vi "oldProceed.vi"(8 "error in (no error)":errorcluster, 11 "DAQMH121119OrcaFlash in":refnum<class "DAQOrcaFlash.lvclass">) -> (0 "error out":errorcluster, 3 "DAQMH121119OrcaFlash out":refnum<class "DAQOrcaFlash.lvclass">)   [LabVIEW 2012]
uses:
  DAQOrcaFlash.lvclass
  Murmex/LabVIEW/Murmex/Murmex/Murmex.lvclass
  Murmex/LabVIEW/Murmex/StopMessage/StopMessage.lvclass
  Murmex/LabVIEW/Murmex/GenericMessage/GenericMessage.lvclass
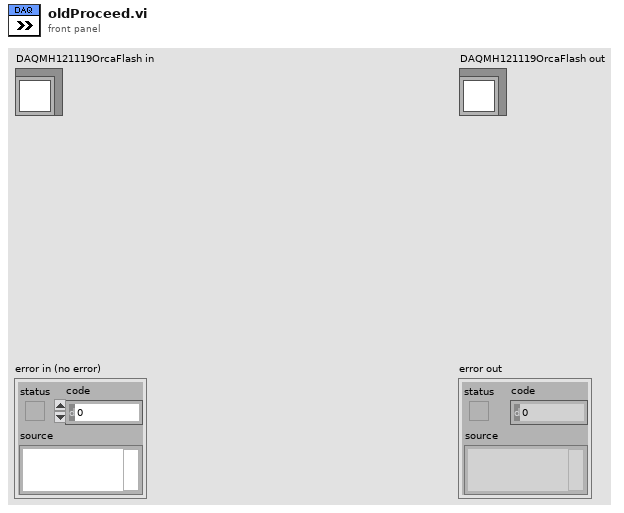
[diagram p1: front panel]
types:
  T1 = typedef "DAQOrcaFlash.lvclass/imaging_mode.ctl" = enum16{"focus mode", "single sweep"}
  T2 = typedef "IMAQ Image.ctl" = refnum<image>
  T3 = cluster{"width":u32, "height":u32, "datatype":u32}
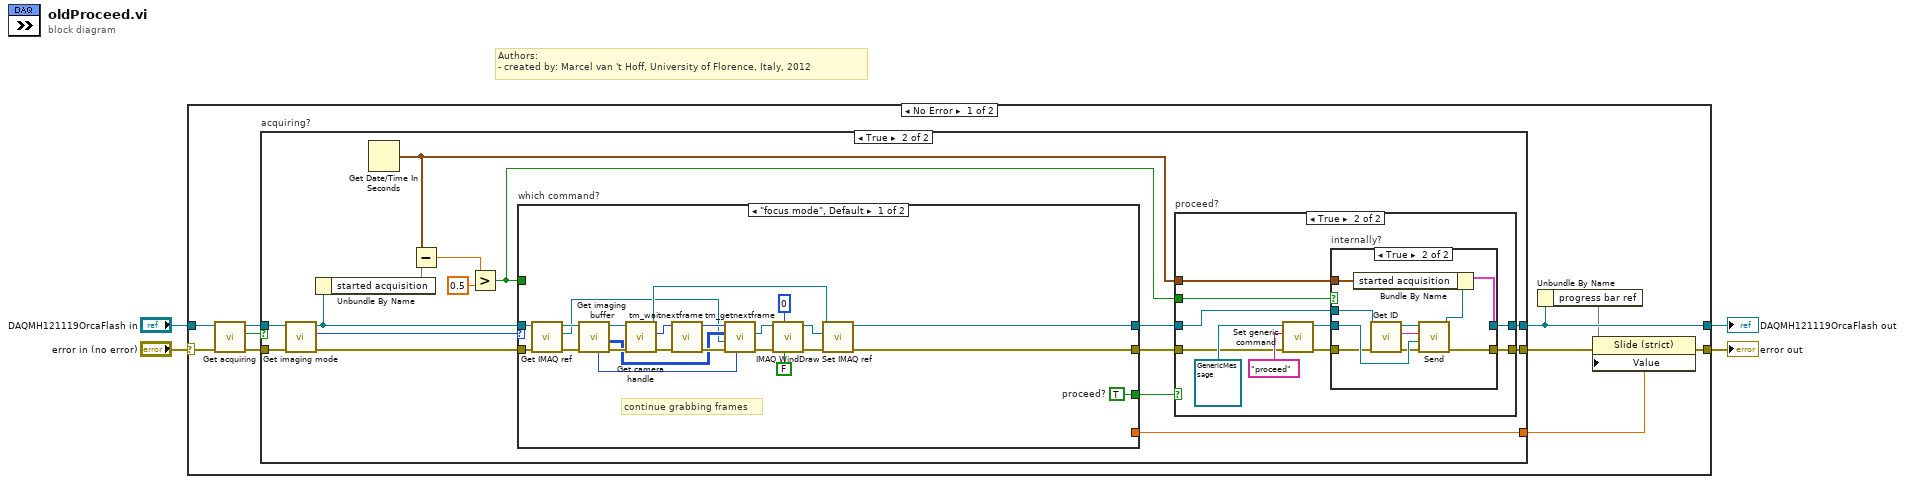
[diagram p0: block diagram]
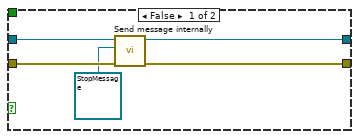
[diagram p3: hidden frame]
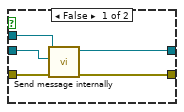
[diagram p4: hidden frame]
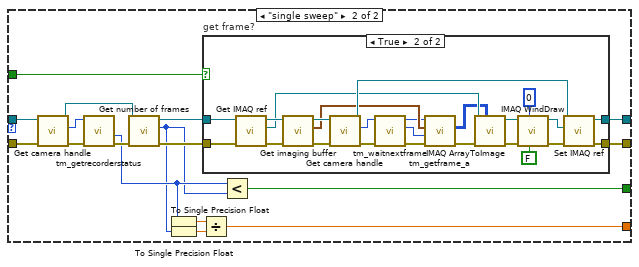
[diagram p5: hidden frame]
diagram:
  # "Authors: \n- created by: Marcel van 't Hoff, University of Florence, Italy, 2012"
  n1 = case shown="No Error" "error in (no error)" {
    selector: "error in (no error)" -> [w12 w130]
    tunnel: [w6 w130] -> w3
    tunnel: [w9 w129] -> w1
    tunnel: "DAQMH121119OrcaFlash in" -> [w14 w129]
    frame No Error {
      n2 = call "Get acquiring.vi"("error in (no error)"=w12, "DAQMH121119OrcaFlash in"=w14) -> ("error out"=w11:errorcluster, "is acquiring?"=w10:bool, "DAQMH121119OrcaFlash out"=w13:refnum<class "DAQOrcaFlash.lvclass">)  [unwired: 7 in]
      n3 = case "acquiring?" shown="True" w10 {
        tunnel: [w15 w24] -> w5
        tunnel: [w16 w25] -> w9
        tunnel: w13 -> [w16 w30]
        tunnel: w11 -> [w15 w29]
        tunnel: [_ w28] -> w7
        frame False {
        }
        frame True {
          n4 = call "Get imaging mode.vi"("error in (no error)"=w29, "DAQMH121119OrcaFlash in"=w30) -> ("error out"=w32:errorcluster, "imaging mode"=w31:T1, "DAQMH121119OrcaFlash out"=w18:refnum<class "DAQOrcaFlash.lvclass">)  [unwired: 7 in]
          n5 = Unbundle By Name(w18) -> ("started acquisition"=w20)
          n6 = Get Date/Time In Seconds() -> (seconds since 1Jan1904=w17:timestamp)
          n7 = Subtract(x=w17, y=w20) -> (x-y=w21:dbl)
          n8 = Greater?(x=w21, y=0.5) -> (0:w19:bool)
          n9 = case "which command?" shown="\"focus mode\", Default" w31 {
            tunnel: w32 -> [w84 w102]
            tunnel: w18 -> [w85 w100]
            tunnel: [w83 w90] -> w27
            tunnel: [w82 w91] -> w26
            tunnel: [_ w92] -> w28
            tunnel: [w81 w86] -> w23
            tunnel: w19 -> [_ w89]
            frame "focus mode", Default {
              w81 = TRUE  # proceed?
              # "continue grabbing frames"
              n10 = call "Get IMAQ ref.vi"("error in (no error)"=w84, "DAQMH121119OrcaFlash in"=w85) -> ("error out"=w74:errorcluster, "IMAQ reference"=w70:T2, "DAQMH121119OrcaFlash out"=w77:refnum<class "DAQOrcaFlash.lvclass">)  [unwired: 7 in]
              n11 = call "Get imaging buffer.vi"("error in (no error)"=w74, "DAQMH121119OrcaFlash in"=w77) -> ("error out"=w73:errorcluster, "Buffer 2"=w71:u16[][], "DAQMH121119OrcaFlash out"=w75:refnum<class "DAQOrcaFlash.lvclass">, "Image type"=w69:u32)  [unwired: 5 in, 1 out]
              n12 = call "Get camera handle.vi"("error in (no error)"=w73, "DAQMH121119OrcaFlash in"=w75) -> ("error out"=w78:errorcluster, "cam handle"=w79:u32, "DAQMH121119OrcaFlash out"=w76:refnum<class "DAQOrcaFlash.lvclass">)  [unwired: 7 in]
              n13 = call <userlib>:"tm_waitnextframe.vi"("error in (no error)"=w78, "Handle in"=w79) -> ("error out"=w80:errorcluster, "Handle out"=w72:u32)  [unwired: 6 in, 2 out]
              n14 = call <userlib>:"tm_getnextframe.vi"("Image Type"=w69, "error in (no error)"=w80, "Image"=w70, "Buffer"=w71, "Handle in"=w72) -> ("error out"=w66:errorcluster, "New Image"=w68:T2)  [unwired: 4 in, 1 out]
              n15 = call "IMAQ WindDraw"("Resize to Image Size? (Y)"=FALSE, "Window Number (0...15)"=0, "error in (no error)"=w66, "Image"=w68) -> ("error out"=w65:errorcluster, "Image Out (duplicate)"=w67:T2)  [unwired: 6 in]
              n16 = call "Set IMAQ ref.vi"("error in (no error)"=w65, "IMAQ reference"=w67, "DAQMH121119OrcaFlash in"=w76) -> ("error out"=w83:errorcluster, "DAQMH121119OrcaFlash out"=w82:refnum<class "DAQOrcaFlash.lvclass">)  [unwired: 7 in]
            }
            frame "single sweep" {
              n17 = call "Get camera handle.vi"("error in (no error)"=w102, "DAQMH121119OrcaFlash in"=w100) -> ("error out"=w101:errorcluster, "cam handle"=w99:u32, "DAQMH121119OrcaFlash out"=w98:refnum<class "DAQOrcaFlash.lvclass">)  [unwired: 7 in]
              n18 = call <userlib>:"tm_getrecorderstatus.vi"("error in (no error)"=w101, "Handle"=w99) -> ("error out"=w97:errorcluster, "Count"=w88:i32)  [unwired: 6 in, 2 out]
              n19 = call "Get number of frames.vi"("error in (no error)"=w97, "DAQMH121119OrcaFlash in"=w98) -> ("error out"=w96:errorcluster, "no. of frames"=w87:i32, "DAQMH121119OrcaFlash out"=w95:refnum<class "DAQOrcaFlash.lvclass">)  [unwired: 7 in]
              n20 = To Single Precision Float(number=w88) -> (single precision float=w93:sgl)
              n21 = To Single Precision Float(number=w87) -> (single precision float=w94:sgl)
              n22 = Divide(x=w93, y=w94) -> (x/y=w92:sgl)
              n23 = case "get frame?" shown="True" w89 {
                tunnel: w96 -> [w104 w120]
                tunnel: w95 -> [w103 w119]
                tunnel: [w103 w117] -> w91
                tunnel: [w104 w118] -> w90
                frame False {
                }
                frame True {
                  n24 = call "Get IMAQ ref.vi"("error in (no error)"=w120, "DAQMH121119OrcaFlash in"=w119) -> ("error out"=w127:errorcluster, "IMAQ reference"=w122:T2, "DAQMH121119OrcaFlash out"=w124:refnum<class "DAQOrcaFlash.lvclass">)  [unwired: 7 in]
                  n25 = call "Get imaging buffer.vi"("error in (no error)"=w127, "DAQMH121119OrcaFlash in"=w124) -> ("error out"=w128:errorcluster, "imaging buffer"=w116:T3, "DAQMH121119OrcaFlash out"=w126:refnum<class "DAQOrcaFlash.lvclass">)  [unwired: 5 in, 2 out]
                  n26 = call "Get camera handle.vi"("error in (no error)"=w128, "DAQMH121119OrcaFlash in"=w126) -> ("error out"=w112:errorcluster, "cam handle"=w115:u32, "DAQMH121119OrcaFlash out"=w125:refnum<class "DAQOrcaFlash.lvclass">)  [unwired: 7 in]
                  n27 = call <userlib>:"tm_waitnextframe.vi"("error in (no error)"=w112, "Handle in"=w115) -> ("error out"=w111:errorcluster, "Frame Index"=w113:i32, "Handle out"=w114:u32)  [unwired: 6 in, 1 out]
                  n28 = call <userlib>:"tm_getframe_a.vi"("error in (no error)"=w111, "Frame Index"=w113, "Buffer"=w116, "Handle in"=w114) -> ("error out"=w123:errorcluster, "Data 16"=w121:u16[][])  [unwired: 3 in, 3 out]
                  n29 = call "IMAQ ArrayToImage"("Image Pixels (U16)"=w121, "error in (no error)"=w123, "Image"=w122) -> ("error out"=w110:errorcluster, "Image Out"=w108:T2)  [unwired: 7 in]
                  n30 = call "IMAQ WindDraw"("Resize to Image Size? (Y)"=FALSE, "Window Number (0...15)"=0, "error in (no error)"=w110, "Image"=w108) -> ("error out"=w109:errorcluster, "Image Out (duplicate)"=w107:T2)  [unwired: 6 in]
                  n31 = call "Set IMAQ ref.vi"("error in (no error)"=w109, "IMAQ reference"=w107, "DAQMH121119OrcaFlash in"=w125) -> ("error out"=w118:errorcluster, "DAQMH121119OrcaFlash out"=w117:refnum<class "DAQOrcaFlash.lvclass">)  [unwired: 7 in]
                }
              }
              n32 = Less?(x=w88, y=w87) -> (x < y?=w86:bool)
            }
          }
          n33 = case "proceed?" shown="True" w23 {
            tunnel: w27 -> [w36 w43]
            tunnel: [w34 w40] -> w24
            tunnel: w26 -> [w37 w42]
            tunnel: [w33 w41] -> w25
            tunnel: w19 -> [_ w39]
            tunnel: w17 -> [_ w38]
            frame False {
              n34 = call "Send message internally.vi"("error in (no error)"=w36, "Message"=refnum<class "StopMessage.lvclass"> refnum ("StopMessage.lvclass"), "Murmex in"=w37) -> ("error out"=w34:errorcluster, "Murmex out"=w33:refnum<class "DAQOrcaFlash.lvclass">)  [unwired: 7 in]
            }
            frame True {
              n35 = call "Set generic command.vi"("error in (no error)"=w43, "generic command"="proceed" ("input string"), "GenericMessage in"=refnum<class "GenericMessage.lvclass"> refnum ("GenericMessage.lvclass")) -> ("error out"=w46:errorcluster, "GenericMessage out"=w45:refnum<class "GenericMessage.lvclass">)  [unwired: 7 in]
              n36 = case "internally?" shown="True" w39 {
                tunnel: w46 -> [w52 w58]
                tunnel: w45 -> [w51 w60]
                tunnel: w42 -> [w50 w61]
                tunnel: [w49 w53] -> w41
                tunnel: [w48 w62] -> w40
                tunnel: w38 -> [_ w55]
                frame False {
                  n37 = call "Send message internally.vi"("error in (no error)"=w52, "Message"=w51, "Murmex in"=w50) -> ("error out"=w48:errorcluster, "Murmex out"=w49:refnum<class "DAQOrcaFlash.lvclass">)  [unwired: 7 in]
                }
                frame True {
                  n38 = call "Get ID.vi"("error in (no error)"=w58, "Murmex in"=w61) -> ("error out"=w57:errorcluster, "component id"=w56:string, "Murmex out"=w59:refnum<class "DAQOrcaFlash.lvclass">)  [unwired: 7 in]
                  n39 = call "Send.vi"("error in (no error)"=w57, "Message"=w60, "recipient"=w56, "Murmex in"=w59) -> ("error out"=w62:errorcluster, "Murmex out"=w54:refnum<class "DAQOrcaFlash.lvclass">)  [unwired: 6 in]
                  n40 = Bundle By Name(cluster=w54, "started acquisition"=w55) -> (w53:cluster{})
                }
              }
            }
          }
        }
      }
      n41 = Unbundle By Name(w9) -> ("progress bar ref"=w8)
      n42 = property class="Slide (strict)"(reference=w8, error in=w5, "Value"=w7) -> (error out=w6:errorcluster)  [unwired: 1 out]
    }
    frame Error {
    }
  }
  "error out" <- w3
  "DAQMH121119OrcaFlash out" <- w1
